vi "ProdaNG.Tree.Selection.GetTS.vi"(7 "TestStepsTree":refnum<vi>, 8 "error in (no error)":errorcluster) -> (0 "error out":errorcluster, 1 "Selected Element":T2, 2 "LastTS":T3, 5 "Eleemnt Type":T1)   [LabVIEW 2016]
uses:
  ProdaNG.Tree.Fglb.Data.ctl
  ProdaNG.Tree.Fglb.Element.ctl
  ProdaNG.Tree.Fglb.Value.ctl
  ProdaNG.Tree.Fglb.Action.ctl
  ProdaNG.Configurator.Glb.vi
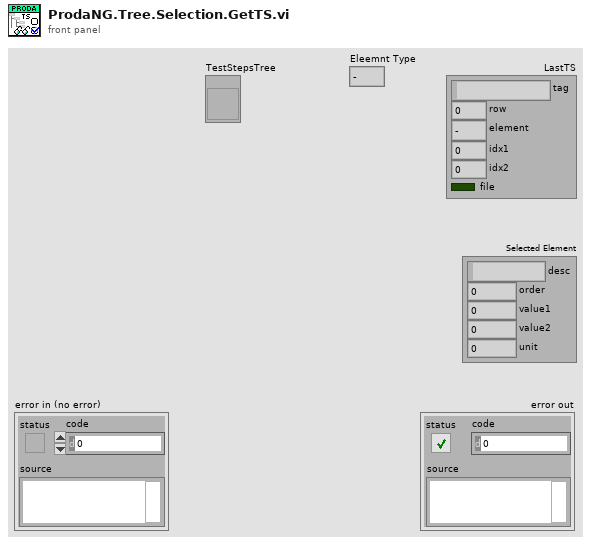
[diagram p1: front panel]
types:
  T1 = typedef "ProdaNG.Tree.Fglb.Element.ctl" = enum16{"-", "PP", "TS", "TP", "TV"}
  T2 = typedef "ProdaNG.Tree.Fglb.Value.ctl" = cluster{"desc":string, "order":i32, "value1":dbl, "value2":dbl, "unit":i32}
  T3 = typedef "ProdaNG.Tree.Fglb.Data.ctl" = cluster{"tag":string, "row":i32, "element":T1, "idx1":i32, "idx2":i32, "file":bool}
  T4 = typedef "ProdaNG.Tree.Fglb.Action.ctl" = enum16{"init", "add", "get by row", "get by tag", "get by idx"}
  T5 = typedef "ProdaNG.ProcessStepParam.ctl" = cluster{"i_id":i32, "processStepId":i32, "unitId":i32, "contentId":string, "previewId":string, "value":dbl, "valueText":string, "paramSequence":i32, "history":i32, "mdReason":string, "mdUser":string, "mdTime":string, "description":string}
  T6 = typedef "ProdaNG.TestStep.ctl" = cluster{"i_id":i32, "processStepId":i32, "testSequence":i32, "testOrder":i32, "mdReason":string, "mdUser":string, "mdTime":string, "description":string}
  T7 = typedef "ProdaNG.TestStepParam.ctl" = cluster{"i_id":i32, "testStepId":i32, "unitId":i32, "contentId":string, "previewId":string, "value":dbl, "valueText":string, "paramSequence":i32, "history":i32, "mdReason":string, "mdUser":string, "mdTime":string, "description":string}
  T8 = typedef "ProdaNG.TestValue.ctl" = cluster{"i_id":i32, "testStepId":i32, "releaseId":i32, "unitId":i32, "contentId":string, "previewId":string, "maximum":dbl, "minimum":dbl, "valueText":string, "testValueSequence":i32, "history":i32, "mdReason":string, "mdUser":string, "mdTime":string, "description":string}
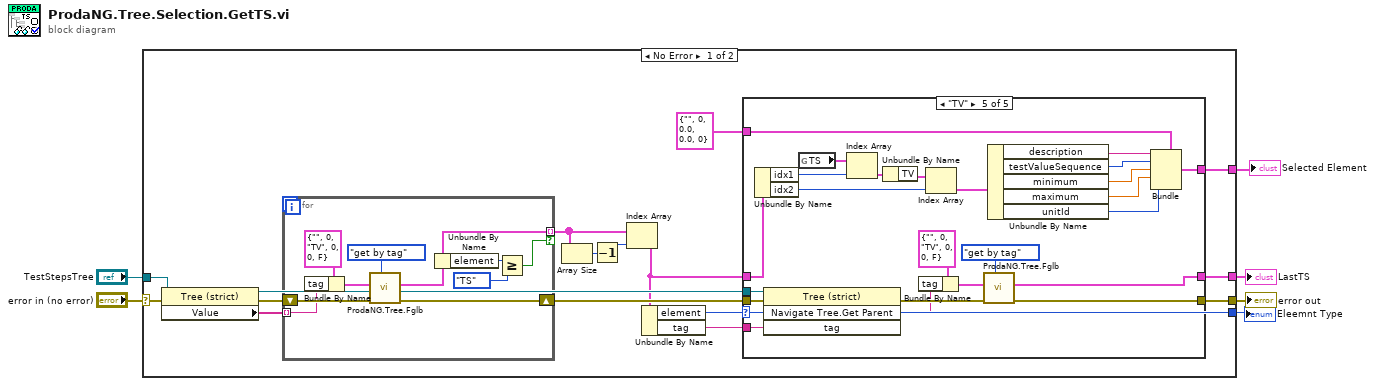
[diagram p0: block diagram]
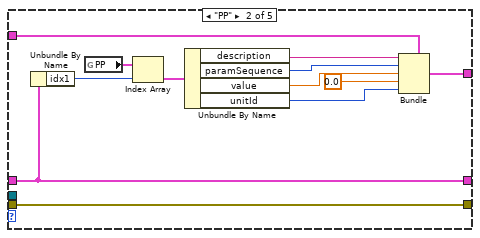
[diagram p3: hidden frame]
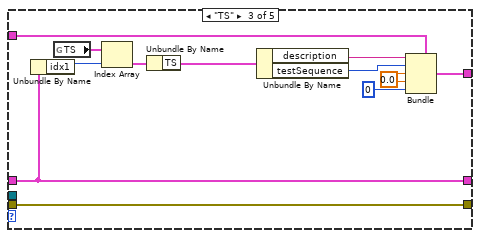
[diagram p4: hidden frame]
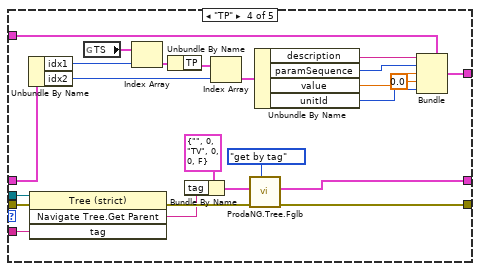
[diagram p5: hidden frame]
diagram:
  n1 = case shown="No Error" "error in (no error)" {
    selector: "error in (no error)" -> [w22 w105]
    tunnel: "TestStepsTree" -> [w20 _]
    tunnel: [w13 w105] -> w6
    tunnel: [w12 _] -> w3
    tunnel: [w8 _] -> w2
    tunnel: [w7 _] -> w1
    frame No Error {
      n2 = property on="Property Node" class="Tree (strict)"(reference=w20, error in=w22) -> (reference out=w14:refnum<vi>, error out=w21:errorcluster, "Value"=w19:string[])
      n3 = for {
        tunnel: w19 -> [w97] mode=indexing
        shift-right: [w100] -> w15
        shift-left: w21 -> [w101]
        tunnel: [w98] -> w16 mode=indexing if=w95
        n4 = Bundle By Name(cluster=T3 {"tag"="", "row"=0, "element"=enum."TV", "idx1"=0, "idx2"=0, "file"=FALSE} ("entry in"), "tag"=w97) -> (w102:T3)
        n5 = call "ProdaNG.Tree.Fglb.vi"("Action (add)"=ProdaNG.Tree.Fglb.Action."get by tag", "error in"=w101, "entry in"=w102) -> ("error out"=w100:errorcluster, "found entry"=w98:T3)  [unwired: 6 in, 1 out]
        n6 = Unbundle By Name(w98) -> ("element"=w99:T1)
        n7 = Greater Or Equal?(x=w99, y=ProdaNG.Tree.Fglb.Element."TS") -> (x >= y?=w95:bool)
      }
      n8 = Array Size(array=w16) -> (size(s)=w18:i32)
      n9 = Decrement(x=w18) -> (x-1=w17:i32)
      n10 = Index Array(array=w16, index=w17) -> (element=w9:T3)
      n11 = Unbundle By Name(w9) -> ("element"=w7:T1, "tag"=w11:string)
      n12 = case shown="\"TV\"" w7 {
        tunnel: w15 -> [w23 w25 w47 w71 w94]
        tunnel: w14 -> [_ _ _ w70 w93]
        tunnel: [w23 w25 w47 w69 w92] -> w13
        tunnel: [w24 w26 w48 w50 w87] -> w12
        tunnel: w11 -> [_ _ _ w64 w86]
        tunnel: [_ w27 w38 w51 w73] -> w8
        tunnel: T2 {"desc"="", "order"=0, "value1"=0.0, "value2"=0.0, "unit"=0} ("Selected Element") -> [_ w28 w37 w49 w72]
        tunnel: w9 -> [w24 w26 w48 w54 w76]
        frame "-" {
        }
        frame "PP" {
          n13 = Unbundle By Name(w26) -> ("idx1"=w29:i32)
          n14 = global read "ProdaNG.Configurator.Glb.vi" "PP"() -> (w36:T5[])
          n15 = Index Array(array=w36, index=w29) -> (element=w33:T5)
          n16 = Unbundle By Name(w33) -> ("description"=w35:string, "paramSequence"=w34:i32, "value"=w32:dbl, "unitId"=w30:i32)
          n17 = Bundle(cluster=w28, "desc"=w35, "order"=w34, "value1"=w32, "value2"=0.0, "unit"=w30) -> (w27:T2)
        }
        frame "TS" {
          w42 = 0.0
          n18 = Unbundle By Name(w48) -> ("idx1"=w39:i32)
          n19 = global read "ProdaNG.Configurator.Glb.vi" "TS"() -> (w46:cluster{"TS":T6, "TP":T7[], "TV":T8[]}[])
          n20 = Index Array(array=w46, index=w39) -> (element=w43:cluster{"TS":T6, "TP":T7[], "TV":T8[]})
          n21 = Unbundle By Name(w43) -> ("TS"=w41:T6)
          n22 = Unbundle By Name(w41) -> ("description"=w45:string, "testSequence"=w44:i32)
          n23 = Bundle(cluster=w37, "desc"=w45, "order"=w44, "value1"=w42, "value2"=w42, "unit"=0 ("unitId")) -> (w38:T2)
        }
        frame "TP" {
          n24 = Unbundle By Name(w54) -> ("idx1"=w53:i32, "idx2"=w52:i32)
          n25 = invoke class="Tree (strict)" method="Navigate Tree.Get Parent"(reference=w70, error in=w71, "tag"=w64) -> (error out=w69:errorcluster, "Navigate Tree:Get Parent"=w65:string)  [unwired: 1 in, 2 out]
          n26 = global read "ProdaNG.Configurator.Glb.vi" "TS"() -> (w63:cluster{"TS":T6, "TP":T7[], "TV":T8[]}[])
          n27 = Index Array(array=w63, index=w53) -> (element=w62:cluster{"TS":T6, "TP":T7[], "TV":T8[]})
          n28 = Unbundle By Name(w62) -> ("TP"=w61:T7[])
          n29 = Bundle By Name(cluster=T3 {"tag"="", "row"=0, "element"=enum."TV", "idx1"=0, "idx2"=0, "file"=FALSE} ("entry in"), "tag"=w65) -> (w68:T3)
          n30 = Index Array(array=w61, index=w52) -> (element=w60:T7)
          n31 = call "ProdaNG.Tree.Fglb.vi"("Action (add)"=ProdaNG.Tree.Fglb.Action."get by tag", "entry in"=w68) -> ("found entry"=w50:T3)  [unwired: 7 in, 2 out]
          n32 = Unbundle By Name(w60) -> ("description"=w59:string, "paramSequence"=w58:i32, "value"=w57:dbl, "unitId"=w55:i32)
          n33 = Bundle(cluster=w49, "desc"=w59, "order"=w58, "value1"=w57, "value2"=0.0, "unit"=w55) -> (w51:T2)
        }
        frame "TV" {
          n34 = Unbundle By Name(w76) -> ("idx1"=w75:i32, "idx2"=w74:i32)
          n35 = invoke class="Tree (strict)" method="Navigate Tree.Get Parent"(reference=w93, error in=w94, "tag"=w86) -> (error out=w92:errorcluster, "Navigate Tree:Get Parent"=w88:string)  [unwired: 1 in, 2 out]
          n36 = global read "ProdaNG.Configurator.Glb.vi" "TS"() -> (w85:cluster{"TS":T6, "TP":T7[], "TV":T8[]}[])
          n37 = Index Array(array=w85, index=w75) -> (element=w84:cluster{"TS":T6, "TP":T7[], "TV":T8[]})
          n38 = Unbundle By Name(w84) -> ("TV"=w83:T8[])
          n39 = Bundle By Name(cluster=T3 {"tag"="", "row"=0, "element"=enum."TV", "idx1"=0, "idx2"=0, "file"=FALSE} ("entry in"), "tag"=w88) -> (w91:T3)
          n40 = Index Array(array=w83, index=w74) -> (element=w82:T8)
          n41 = call "ProdaNG.Tree.Fglb.vi"("Action (add)"=ProdaNG.Tree.Fglb.Action."get by tag", "entry in"=w91) -> ("found entry"=w87:T3)  [unwired: 7 in, 2 out]
          n42 = Unbundle By Name(w82) -> ("description"=w81:string, "testValueSequence"=w80:i32, "minimum"=w79:dbl, "maximum"=w78:dbl, "unitId"=w77:i32)
          n43 = Bundle(cluster=w72, "desc"=w81, "order"=w80, "value1"=w79, "value2"=w78, "unit"=w77) -> (w73:T2)
        }
      }
    }
    frame Error {
    }
  }
  "error out" <- w6
  "LastTS" <- w3
  "Selected Element" <- w2
  "Eleemnt Type" <- w1
